vi "LS372_write_only.vi"(11 "File Reference":refnum<file>) -> ()   [LabVIEW 2019]
uses:
  Instrument_Setup.vi
  Global/Global Variables/global.vi
  Global/Global Variables/Data_Display_global.vi
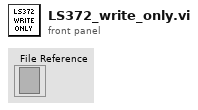
[diagram p1: front panel]
types:
  T1 = typedef "LS372_read_only-Cluster.ctl" = cluster{"LS372-T1":dbl, "LS372 -T2":dbl, "LS372-T4":dbl, "LS372-T5":dbl, "LS372-T6":dbl, "LS372-R1 ":dbl, "LS372-R2":dbl, "LS372-R3 ":dbl, "LS372-R4 \n\n\n\n":dbl, "LS372-R5":dbl, "LS372-R6 ":dbl, "LS372-T3":dbl, "Update Lakeshores":bool}
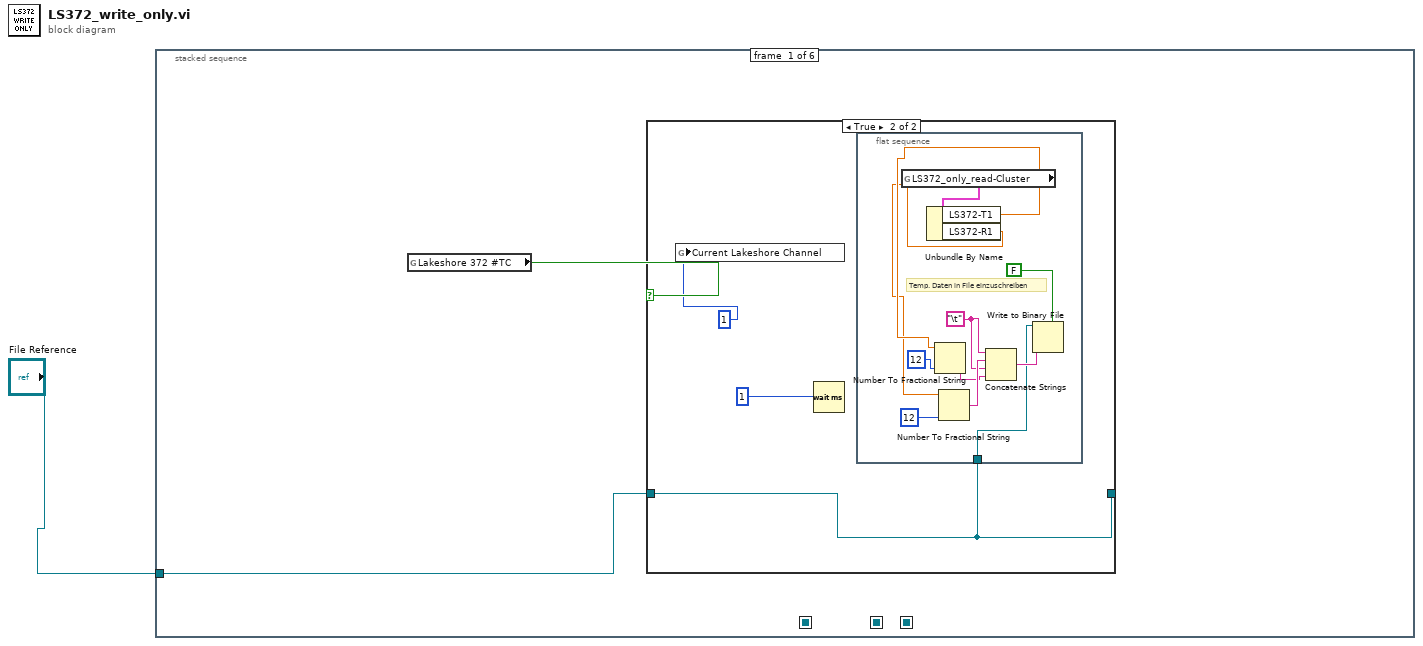
[diagram p0: block diagram]
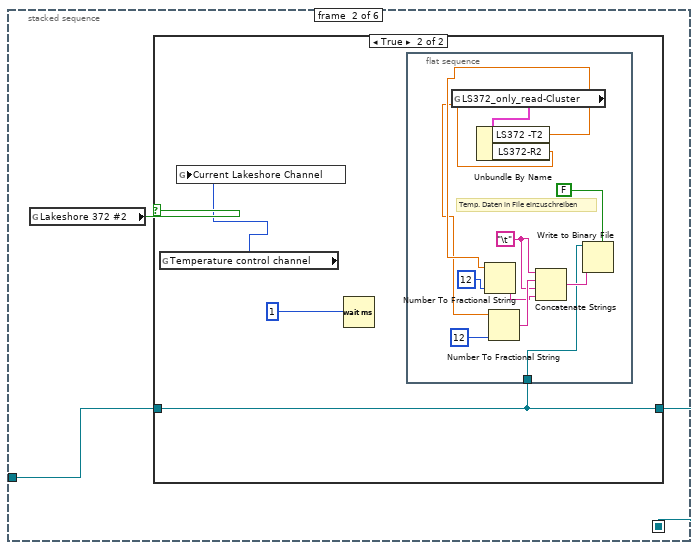
[diagram p3: hidden frame]
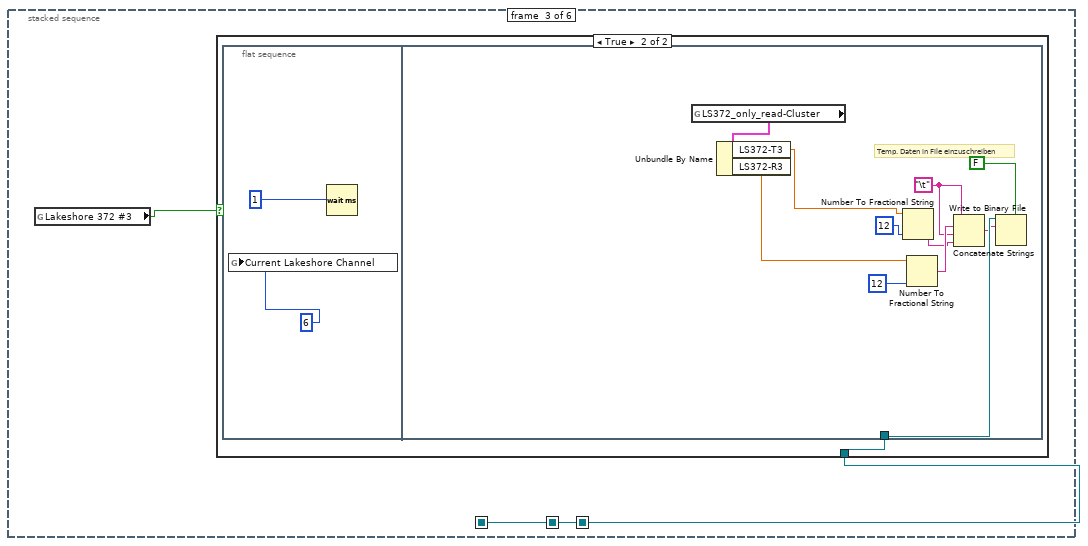
[diagram p5: hidden frame]
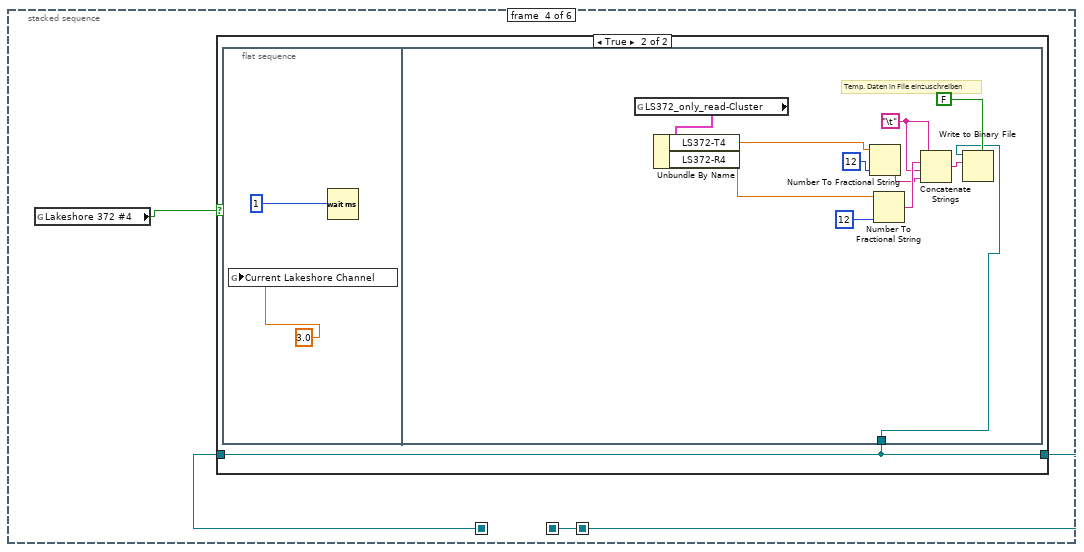
[diagram p7: hidden frame]
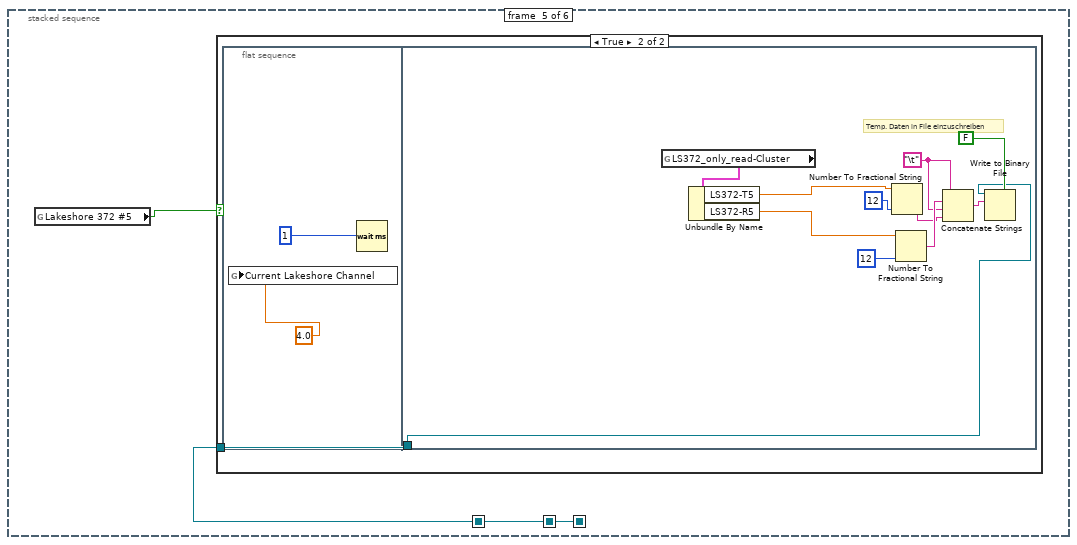
[diagram p9: hidden frame]
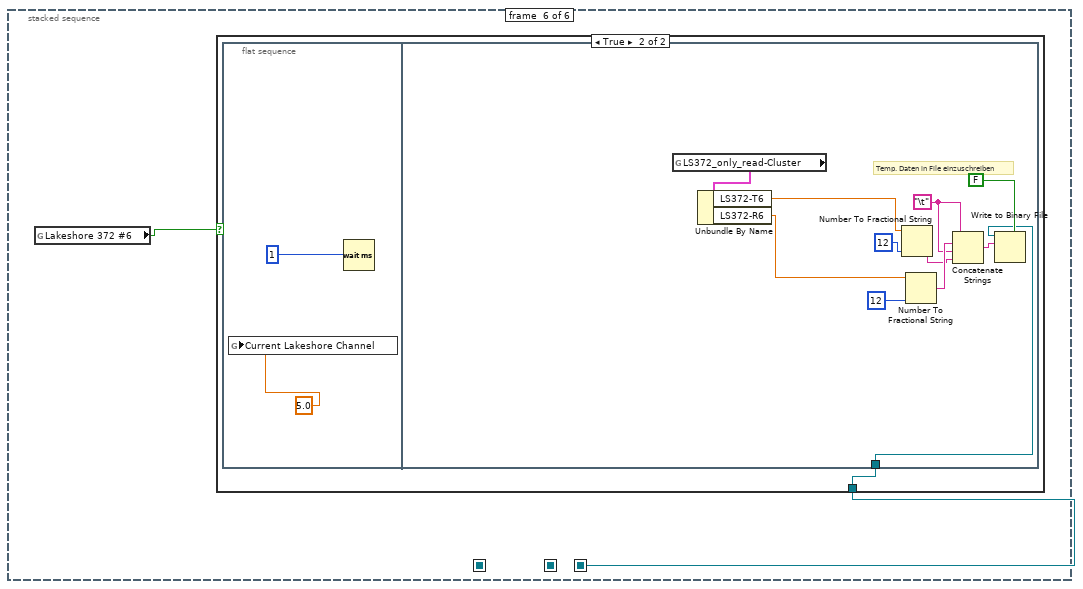
[diagram p11: hidden frame]
diagram:
  n1 = stacked-sequence {
    seq-local: [_ w20 _ _ _ _] -> [_ _ w37 w54 _ _]
    seq-local: [_ _ _ w53 _ _] -> [_ _ _ _ w71 _]
    seq-local: [_ _ _ _ w71 _] -> [_ _ _ _ _ w87]
    tunnel: "File Reference" -> [w2 w19 _ _ _ _]
    frame #0 {
      n2 = global read "Instrument_Setup.vi" "Lakeshore 372 #TC"() -> (w3:bool)
      n3 = case shown="True" w3 {
        tunnel: w2 -> [w4 w5]
        tunnel: [w4 w5] -> _
        frame False {
        }
        frame True {
          n4 = global write "global.vi" "Current Lakeshore Channel"(1) -> ()
          n5 = Wait (ms)(milliseconds to wait=1) -> ()  [unwired: 1 out]
          n6 = flat-sequence {
            tunnel: w5 -> [w11]
            frame #0 {
              w13 = "\t"
              # "Temp. Daten in File einzuschreiben"
              n7 = global read "Data_Display_global.vi" "LS372_only_read-Cluster"() -> (w10:T1)
              n8 = Unbundle By Name(w10) -> ("LS372-T1"=w9:dbl, "LS372-R1"=w8:dbl)
              n9 = Number To Fractional String(number=w9, precision (6)=i16 12) -> (F-format string=w12:string)  [unwired: 2 in]
              n10 = Number To Fractional String(number=w8, precision (6)=i16 12) -> (F-format string=w17:string)  [unwired: 2 in]
              n11 = Concatenate Strings(w13, w17, w13, w12) -> (w18:string)
              n12 = Write to Binary File ("Write File")(file (use dialog)=w11, data=w18, 5:FALSE ("prepend array or string size? (T)")) -> ()  [unwired: 3 in, 3 out]
            }
          }
        }
      }
    }
    frame #1 {
      n13 = global read "Instrument_Setup.vi" "Lakeshore 372 #2"() -> (w21:bool)
      n14 = case shown="True" w21 {
        tunnel: w19 -> [w22 w24]
        tunnel: [w22 w24] -> w20
        frame False {
        }
        frame True {
          n15 = global read "Instrument_Setup.vi" "Temperature control channel"() -> (w23:i32)
          n16 = global write "global.vi" "Current Lakeshore Channel"(w23) -> ()
          n17 = Wait (ms)(milliseconds to wait=1) -> ()  [unwired: 1 out]
          n18 = flat-sequence {
            tunnel: w24 -> [w29]
            frame #0 {
              w31 = "\t"
              # "Temp. Daten in File einzuschreiben"
              n19 = global read "Data_Display_global.vi" "LS372_only_read-Cluster"() -> (w28:T1)
              n20 = Unbundle By Name(w28) -> ("LS372 -T2"=w27:dbl, "LS372-R2"=w26:dbl)
              n21 = Number To Fractional String(number=w27, precision (6)=i16 12) -> (F-format string=w30:string)  [unwired: 2 in]
              n22 = Number To Fractional String(number=w26, precision (6)=i16 12) -> (F-format string=w35:string)  [unwired: 2 in]
              n23 = Concatenate Strings(w31, w35, w31, w30) -> (w36:string)
              n24 = Write to Binary File ("Write File")(file (use dialog)=w29, data=w36, 5:FALSE ("prepend array or string size? (T)")) -> ()  [unwired: 3 in, 3 out]
            }
          }
        }
      }
    }
    frame #2 {
      n25 = global read "Instrument_Setup.vi" "Lakeshore 372 #3"() -> (w38:bool)
      n26 = case shown="True" w38 {
        tunnel: w37 -> [_ w39]
        frame False {
        }
        frame True {
          n27 = flat-sequence {
            tunnel: w39 -> [w51]
            frame #0 {
              n28 = global write "global.vi" "Current Lakeshore Channel"(6) -> ()
              n29 = Wait (ms)(milliseconds to wait=1) -> ()  [unwired: 1 out]
            }
            frame #1 {
              w47 = "\t"
              # "Temp. Daten in File einzuschreiben"
              n30 = global read "Data_Display_global.vi" "LS372_only_read-Cluster"() -> (w44:T1)
              n31 = Unbundle By Name(w44) -> ("LS372-T3"=w43:dbl, "LS372-R3"=w42:dbl)
              n32 = Number To Fractional String(number=w43, precision (6)=i16 12) -> (F-format string=w46:string)  [unwired: 2 in]
              n33 = Number To Fractional String(number=w42, precision (6)=i16 12) -> (F-format string=w50:string)  [unwired: 2 in]
              n34 = Concatenate Strings(w47, w50, w47, w46) -> (w45:string)
              n35 = Write to Binary File ("Write File")(file (use dialog)=w51, data=w45, 5:FALSE ("prepend array or string size? (T)")) -> ()  [unwired: 3 in, 3 out]
            }
          }
        }
      }
    }
    frame #3 {
      n36 = global read "Instrument_Setup.vi" "Lakeshore 372 #4"() -> (w55:bool)
      n37 = case shown="True" w55 {
        tunnel: w54 -> [w56 w57]
        tunnel: [w56 w57] -> w53
        frame False {
        }
        frame True {
          n38 = flat-sequence {
            tunnel: w57 -> [w63]
            frame #0 {
              n39 = global write "global.vi" "Current Lakeshore Channel"(3.0) -> ()
              n40 = Wait (ms)(milliseconds to wait=1) -> ()  [unwired: 1 out]
            }
            frame #1 {
              w66 = "\t"
              # "Temp. Daten in File einzuschreiben"
              n41 = global read "Data_Display_global.vi" "LS372_only_read-Cluster"() -> (w62:T1)
              n42 = Unbundle By Name(w62) -> ("LS372-T4"=w61:dbl, "LS372-R4"=w60:dbl)
              n43 = Number To Fractional String(number=w61, precision (6)=i16 12) -> (F-format string=w65:string)  [unwired: 2 in]
              n44 = Number To Fractional String(number=w60, precision (6)=i16 12) -> (F-format string=w69:string)  [unwired: 2 in]
              n45 = Concatenate Strings(w66, w69, w66, w65) -> (w64:string)
              n46 = Write to Binary File ("Write File")(file (use dialog)=w63, data=w64, 5:FALSE ("prepend array or string size? (T)")) -> ()  [unwired: 3 in, 3 out]
            }
          }
        }
      }
    }
    frame #4 {
      n47 = global read "Instrument_Setup.vi" "Lakeshore 372 #5"() -> (w72:bool)
      n48 = case shown="True" w72 {
        tunnel: w71 -> [_ w73]
        frame False {
        }
        frame True {
          n49 = flat-sequence {
            tunnel: w73 -> [w79]
            frame #0 {
              n50 = global write "global.vi" "Current Lakeshore Channel"(4.0) -> ()
              n51 = Wait (ms)(milliseconds to wait=1) -> ()  [unwired: 1 out]
            }
            frame #1 {
              w82 = "\t"
              # "Temp. Daten in File einzuschreiben"
              n52 = global read "Data_Display_global.vi" "LS372_only_read-Cluster"() -> (w78:T1)
              n53 = Unbundle By Name(w78) -> ("LS372-T5"=w77:dbl, "LS372-R5"=w76:dbl)
              n54 = Number To Fractional String(number=w77, precision (6)=i16 12) -> (F-format string=w81:string)  [unwired: 2 in]
              n55 = Number To Fractional String(number=w76, precision (6)=i16 12) -> (F-format string=w85:string)  [unwired: 2 in]
              n56 = Concatenate Strings(w82, w85, w82, w81) -> (w80:string)
              n57 = Write to Binary File ("Write File")(file (use dialog)=w79, data=w80, 5:FALSE ("prepend array or string size? (T)")) -> ()  [unwired: 3 in, 3 out]
            }
          }
        }
      }
    }
    frame #5 {
      n58 = global read "Instrument_Setup.vi" "Lakeshore 372 #6"() -> (w88:bool)
      n59 = case shown="True" w88 {
        tunnel: w87 -> [_ w89]
        frame False {
        }
        frame True {
          n60 = flat-sequence {
            tunnel: w89 -> [w95]
            frame #0 {
              n61 = global write "global.vi" "Current Lakeshore Channel"(5.0) -> ()
              n62 = Wait (ms)(milliseconds to wait=1) -> ()  [unwired: 1 out]
            }
            frame #1 {
              w98 = "\t"
              # "Temp. Daten in File einzuschreiben"
              n63 = global read "Data_Display_global.vi" "LS372_only_read-Cluster"() -> (w94:T1)
              n64 = Unbundle By Name(w94) -> ("LS372-T6"=w93:dbl, "LS372-R6"=w92:dbl)
              n65 = Number To Fractional String(number=w93, precision (6)=i16 12) -> (F-format string=w97:string)  [unwired: 2 in]
              n66 = Number To Fractional String(number=w92, precision (6)=i16 12) -> (F-format string=w101:string)  [unwired: 2 in]
              n67 = Concatenate Strings(w98, w101, w98, w97) -> (w96:string)
              n68 = Write to Binary File ("Write File")(file (use dialog)=w95, data=w96, 5:FALSE ("prepend array or string size? (T)")) -> ()  [unwired: 3 in, 3 out]
            }
          }
        }
      }
    }
  }
